vi "20220107_Main.vi"() -> ()   [LabVIEW 2019]
panel:
  out "XY Graph":cluster{dbl[], dbl[]}[](graph)
  in  "Stop":bool
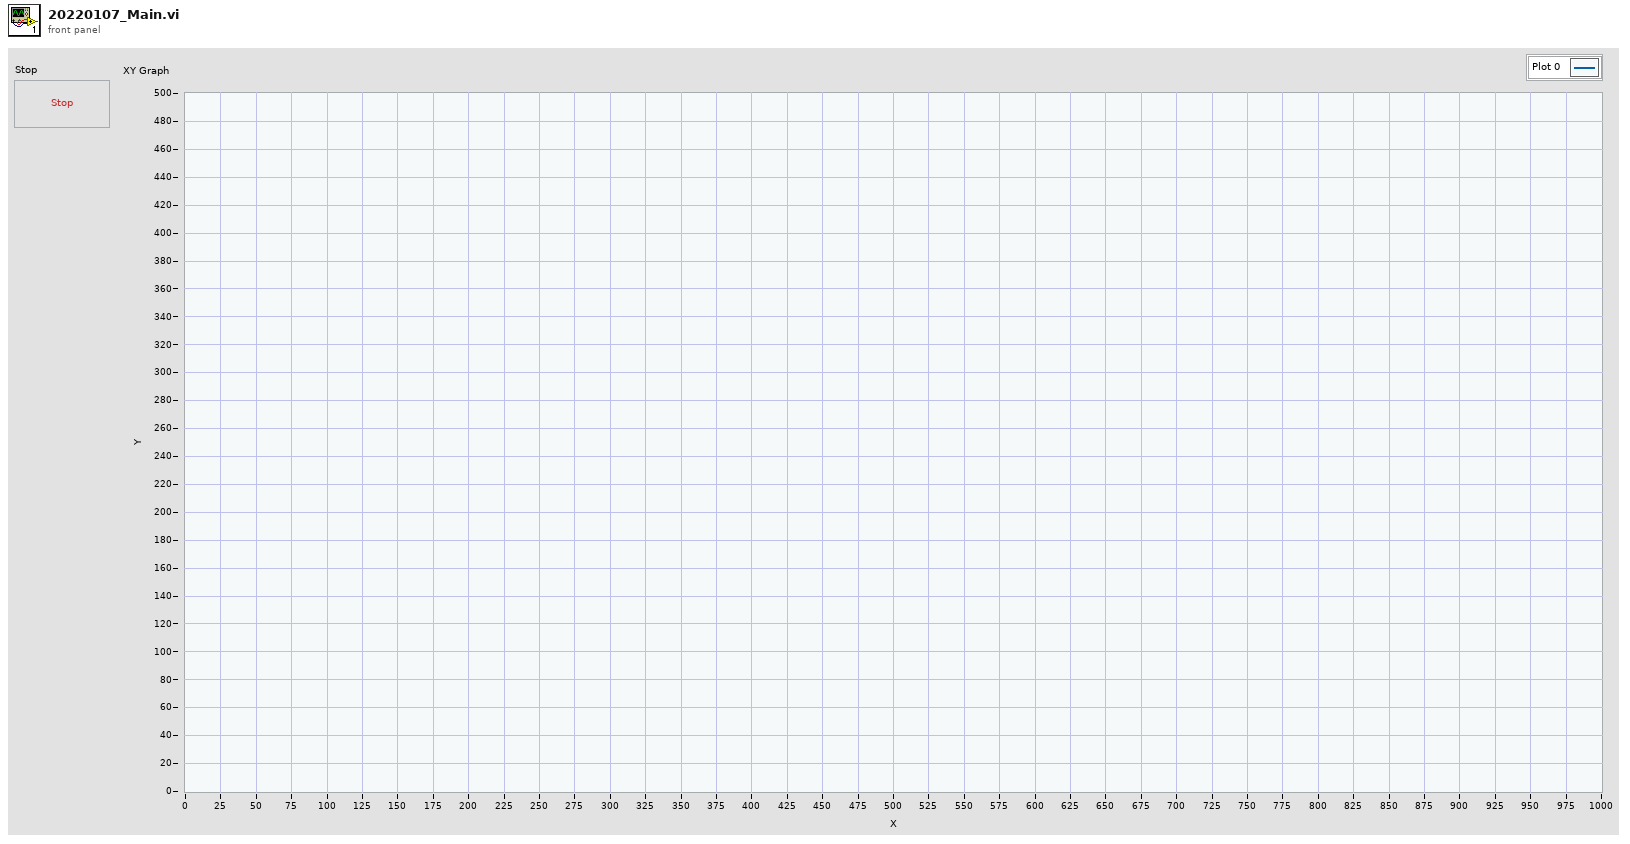
[diagram p1: front panel]
types:
  T1 = typedef "LVPoint32TypeDef.ctl" = cluster{"Horizontal":i32, "Vertical":i32}
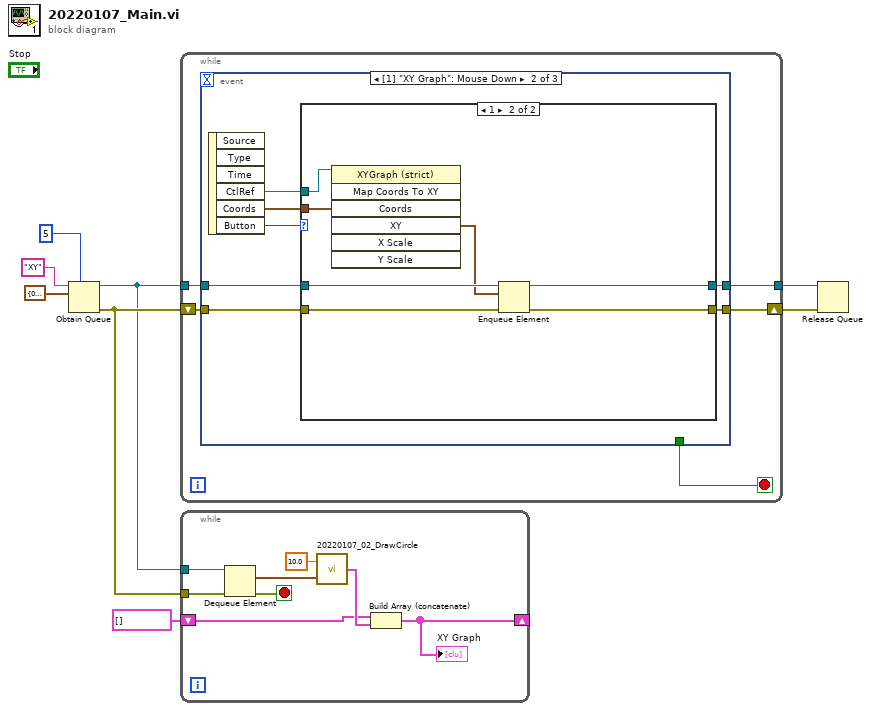
[diagram p0: block diagram]
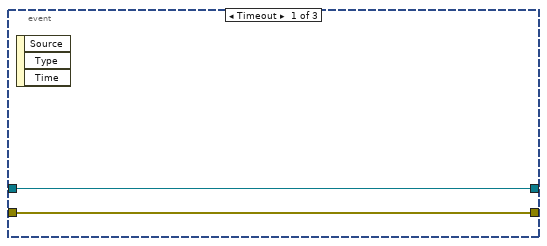
[diagram p2: hidden frame]
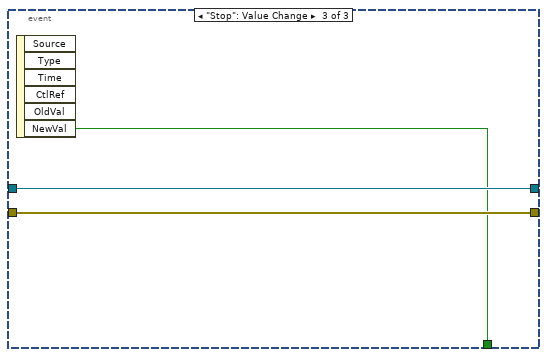
[diagram p4: hidden frame]
diagram:
  n1 = Obtain Queue(max queue size (-1, unlimited)=5, name (unnamed)="XY", element data type=cluster{"X":dbl, "Y":dbl} {"X"=0.0, "Y"=0.0} ("XY")) -> (queue out=w3:refnum<queue>, error out=w4:errorcluster)  [unwired: 2 in, 1 out]
  n2 = while {
    shift-right: [w10] -> w7
    shift-left: w4 -> [w12]
    tunnel: w3 -> [w13]
    tunnel: [w9] -> w6
    stop <- w11 stop-if-true
    n3 = event shown="[1] \"XY Graph\": Mouse Down" {
      selector: _ -> [_ _ _]
      dyn-events: _ -> [_ _ _]
      timeout: _ -> [_ _ _]
      tunnel: w13 -> [w14 w21 w33]
      tunnel: w12 -> [w15 w20 w34]
      tunnel: [w15 w19 w34] -> w10
      tunnel: [w14 w18 w33] -> w9
      tunnel: [_ _ w32] -> w11
      event Timeout {
        n4 = event-data() -> ()  [unwired: 1 in, 3 out]
      }
      event "XY Graph": Mouse Down {
        n5 = event-data() -> ("CtlRef"=w17:refnum<vi>, "Coords"=w16:T1, "Button"=w22:u16)  [unwired: 1 in, 3 out]
        n6 = case shown="1" w22 {
          tunnel: w21 -> [w23 w31]
          tunnel: w20 -> [w24 w30]
          tunnel: [w24 w29] -> w19
          tunnel: [w23 w28] -> w18
          tunnel: w17 -> [_ w27]
          tunnel: w16 -> [_ w26]
          frame 0, Default {
          }
          frame 1 {
            n7 = invoke class="XYGraph (strict)" method="Map Coords To XY"(reference=w27, "Coords"=w26) -> ("XY"=w25:cluster{"X":dbl, "Y":dbl})  [unwired: 5 in, 6 out]
            n8 = Enqueue Element(queue=w31, element=w25, error in (no error)=w30) -> (queue out=w28:refnum<queue>, error out=w29:errorcluster)  [unwired: 1 in, 1 out]
          }
        }
      }
      event "Stop": Value Change {
        n9 = event-data() -> ("NewVal"=w32:bool)  [unwired: 1 in, 5 out]
      }
    }
  }
  n10 = while {
    tunnel: w4 -> [w42]
    tunnel: w3 -> [w41]
    shift-right: [w35] -> _
    shift-left: cluster{dbl[], dbl[]}[] [] -> [w36]
    stop <- w40 stop-if-true
    n11 = Dequeue Element(queue=w41, error in (no error)=w42) -> (element=w39:cluster{"X":dbl, "Y":dbl}, error out=w40:errorcluster)  [unwired: 1 in, 2 out]
    n12 = call "20220107_02_DrawCircle.vi"("Offset"=w39, "Radius"=10.0) -> ("XY Graph"=w37:cluster{dbl[], dbl[]})
    n13 = Build Array (concatenate)(w36, w37) -> (w35:cluster{dbl[], dbl[]}[])
    "XY Graph" <- w35
  }
  n14 = Release Queue(queue=w6, error in (no error)=w7) -> ()  [unwired: 1 in, 3 out]
